vi "ReadAll.vi"(0 "object in":refnum<class "CoriFlowBFS1Plus.lvclass">, 5 "error in (no error)":errorcluster) -> (14 "object out":refnum<class "CoriFlowBFS1Plus.lvclass">, 16 "Coriolis Data":T1, 19 "error out":errorcluster)   [LabVIEW 2021, in "CoriFlowBFS1Plus.lvclass"]
uses:
  CoriFlowBFS1Plus.lvclass
  CoriFlowBFS1Plus.lvclass/CoriFlowBFS1Plus.ctl
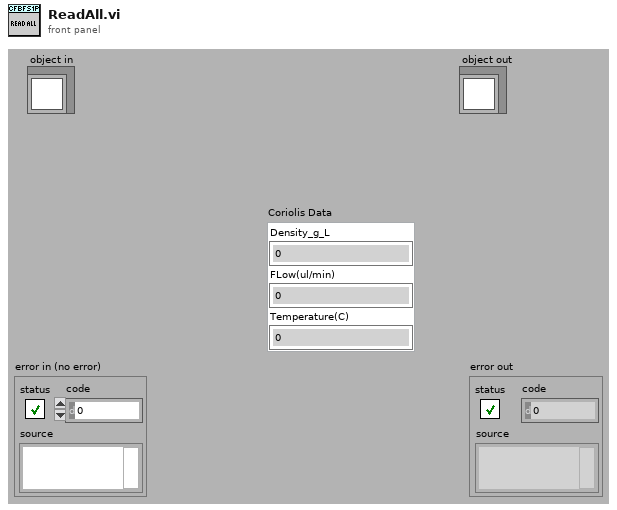
[diagram p1: front panel]
types:
  T1 = cluster{"Density_g_L":sgl, "FLow(ul/min)":sgl, "Temperature(C)":sgl}
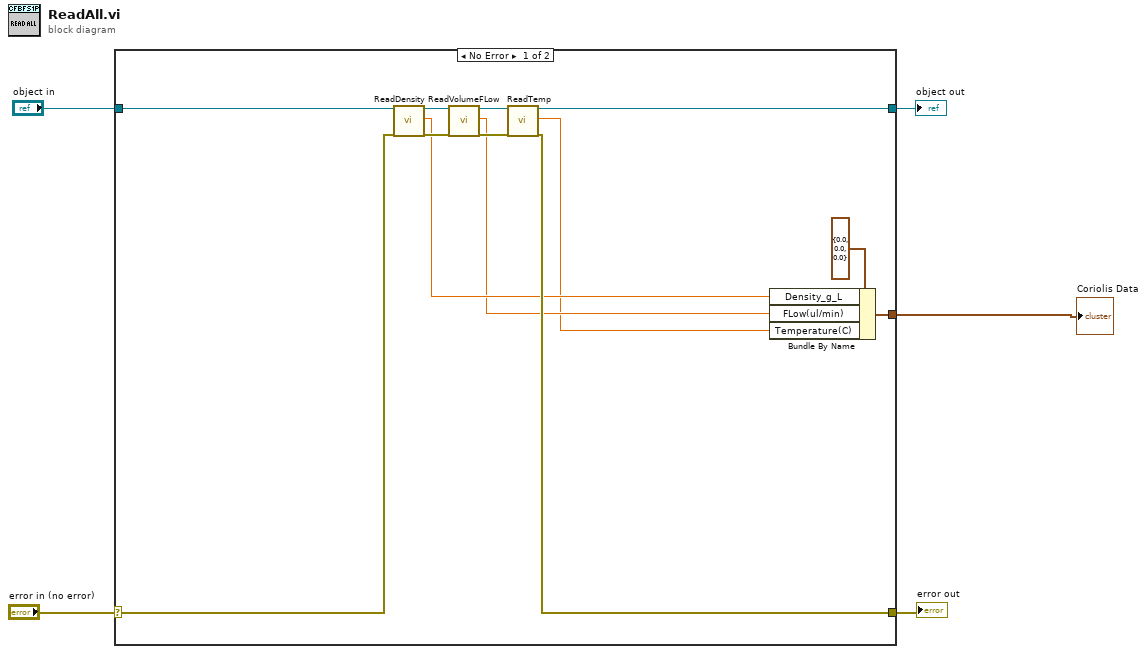
[diagram p0: block diagram]
diagram:
  n1 = case shown="No Error" "error in (no error)" {
    selector: "error in (no error)" -> [w11 w20]
    tunnel: [w12 w20] -> w4
    tunnel: [w16 w19] -> w2
    tunnel: "object in" -> [w15 w19]
    tunnel: [w6 _] -> w1
    frame No Error {
      n2 = call-dynamic "ReadDensity.vi"("object in"=w15, "error in (no error)"=w11) -> ("object out"=w18:refnum<class "CoriFlowBFS1Plus.lvclass">, "Density_g_L"=w9:sgl, "error out"=w14:errorcluster)  [unwired: 15 in]
      n3 = call-dynamic "ReadVolumeFLow.vi"("object in"=w18, "error in (no error)"=w14) -> ("object out"=w17:refnum<class "CoriFlowBFS1Plus.lvclass">, "FLow(ul/min)"=w8:sgl, "error out"=w13:errorcluster)  [unwired: 15 in]
      n4 = call-dynamic "ReadTemp.vi"("object in"=w17, "error in (no error)"=w13) -> ("object out"=w16:refnum<class "CoriFlowBFS1Plus.lvclass">, "Temperature(C)"=w7:sgl, "error out"=w12:errorcluster)  [unwired: 15 in]
      n5 = Bundle By Name(cluster=T1 {"Density_g_L"=0.0, "FLow(ul/min)"=0.0, "Temperature(C)"=0.0} ("Cluster"), "Density_g_L"=w9, "FLow(ul/min)"=w8, "Temperature(C)"=w7) -> (w6:T1)
    }
    frame Error {
    }
  }
  "error out" <- w4
  "object out" <- w2
  "Coriolis Data" <- w1
